vi "Restore.vi"(8 "error in (no error)":errorcluster, 9 "Previous Version":T1, 10 "Data":string, 11 "Static Path Selector in":refnum<class "MGI Static Path Selector.lvclass">) -> (0 "error out":errorcluster, 3 "Static Path Selector out":refnum<class "MGI Static Path Selector.lvclass">)   [LabVIEW 2020, in "MGI Static Path Selector.lvclass"]
uses:
  <userlib>/_MGI/User Interface/Path Selector XControl/Class Hierarchy/Static File Selector/MGI Static Path Selector.lvclass
  <vilib>/_xctls/Version.ctl
  <userlib>/_MGI/User Interface/Path Selector XControl/Class Hierarchy/Static File Selector/MGI Static Path Selector.lvclass/MGI Static Path Selector.ctl
  <userlib>/_MGI/User Interface/Path Selector XControl/Class Hierarchy/MGI Path Selector.lvclass
  <vilib>/Utility/VariantDataType/VariantType.lvlib
  <vilib>/_xctls/XControlSupport.lvlib
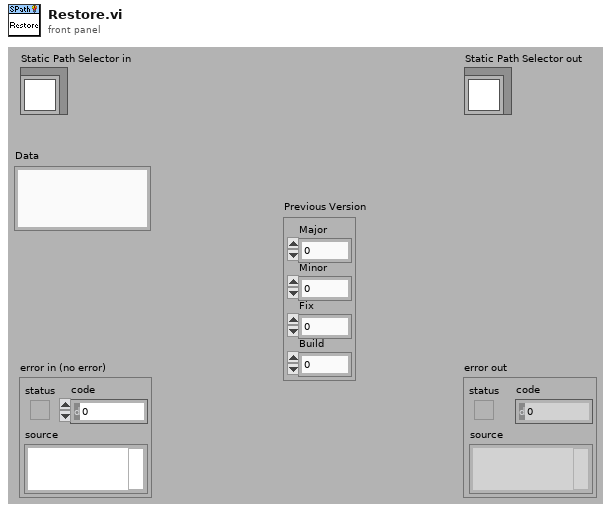
[diagram p1: front panel]
types:
  T1 = typedef "XControlSupport.lvlib/Version.ctl" = cluster{"Major":u16, "Minor":u16, "Fix":u16, "Build":u16}
  T2 = typedef "MGI Static Path Selector.lvclass/Persistent Data Cluster.ctl" = cluster{"Path":path, "Select Option?":bool, "Explorer Option?":bool, "Recurse?":bool, "Allow New?":bool, "Filter":string}
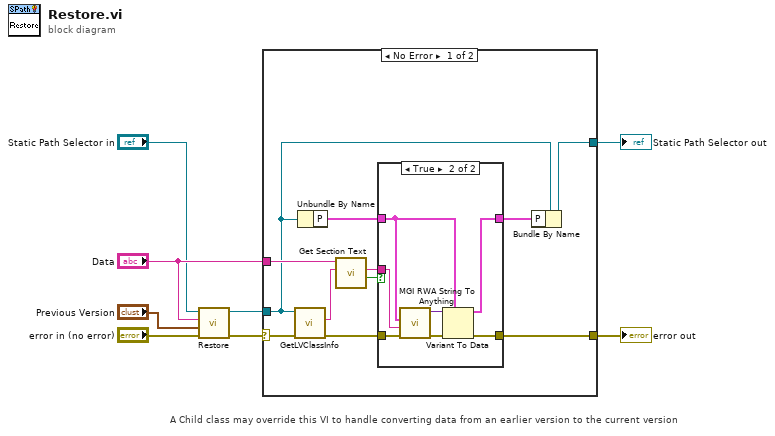
[diagram p0: block diagram]
diagram:
  # "A Child class may override this VI to handle converting data from an earlier version to the current version"
  n1 = call-parent "Restore.vi"("error in (no error)"="error in (no error)", "Previous Version"="Previous Version", "Data"="Data", "Path Selector in"="Static Path Selector in") -> ("error out"=w3:errorcluster, "Path Selector out"=w1:refnum<class "MGI Static Path Selector.lvclass">)  [unwired: 6 in]
  n2 = case shown="No Error" w3 {
    selector: w3 -> [w11 w30]
    tunnel: [w9 w30] -> w8
    tunnel: [w14 w29] -> w7
    tunnel: w1 -> [w10 w29]
    tunnel: "Data" -> [w15 _]
    frame No Error {
      n3 = call <vilib>:"GetLVClassInfo.vi"("error in (no error)"=w11, "Variant"=w10) -> ("error out"=w19:errorcluster, "LV Class File Name"=w18:string)  [unwired: 7 in, 1 out]
      n4 = Unbundle By Name(w10) -> ("P"=w13:T2)
      n5 = call <userlib>:"Get Section Text.vi"("Section Name"=w18, "Data"=w15) -> ("Section Found?"=w16:bool, "Section Text"=w17:string)  [unwired: 8 in]
      n6 = case shown="True" w16 {
        tunnel: w19 -> [w21 w26]
        tunnel: [w21 w25] -> w9
        tunnel: w17 -> [_ w24]
        tunnel: w13 -> [w20 w23]
        tunnel: [w20 w22] -> w12
        frame False {
        }
        frame True {
          n7 = call <userlib>:"MGI RWA String To Anything.vi"("Error In"=w26, "String"=w24, "Type of Anything"=w23) -> ("Error Out"=w27:errorcluster, "Variant"=w28:variant)  [unwired: 6 in, 1 out]
          n8 = Variant To Data(error in=w27, type=w23, Variant=w28) -> (data=w22:T2, error out=w25:errorcluster)
        }
      }
      n9 = Bundle By Name(cluster=w10, "P"=w12) -> (w14:refnum<class "MGI Static Path Selector.lvclass">)
    }
    frame Error {
    }
  }
  "error out" <- w8
  "Static Path Selector out" <- w7
